vi "ExampleSubEvent.vi"(7 "error in (no error)":errorcluster, 8 "Stop Button event source":refnum<vi>, 10 "Button Array event source":refnum<vi>[](array[refnum])) -> (0 "error out":errorcluster)   [LabVIEW 2020]
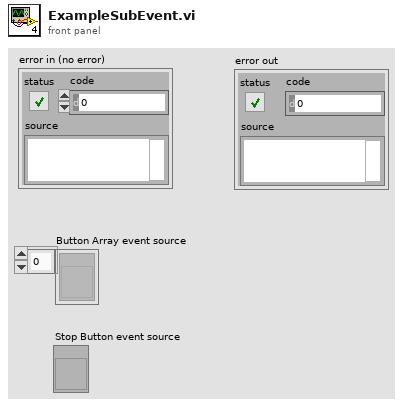
[diagram p1: front panel]
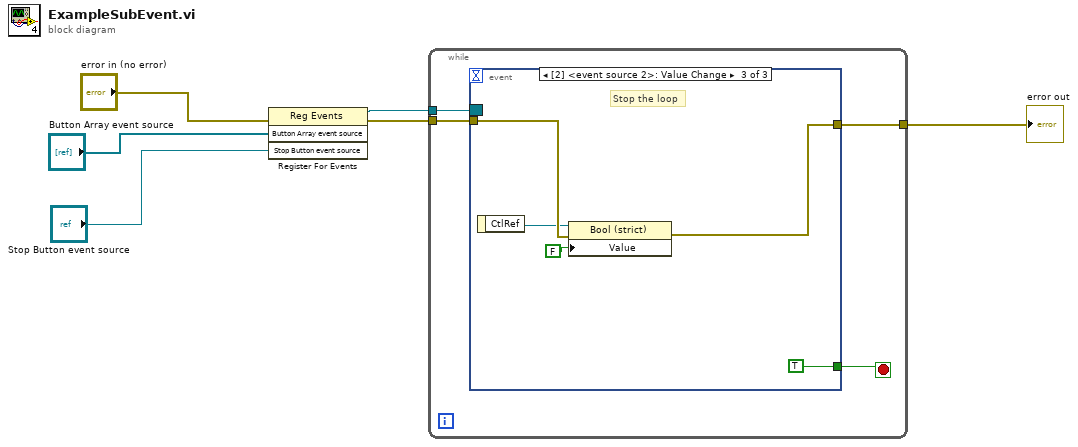
[diagram p0: block diagram]
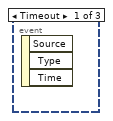
[diagram p2: hidden frame]
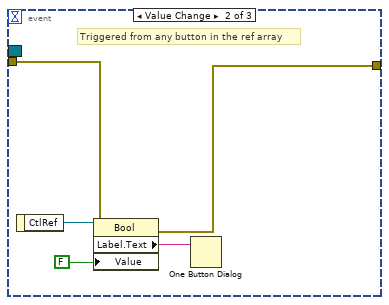
[diagram p3: hidden frame]
diagram:
  n1 = register-events(error in="error in (no error)", "Button Array event source", "Stop Button event source") -> (reference out=w6:refnum<event-registration>, error out=w5:errorcluster)  [unwired: 1 in]
  n2 = while {
    tunnel: w6 -> [w10]
    tunnel: w5 -> [w9]
    tunnel: [w8] -> w4
    stop <- w7 stop-if-true
    n3 = event shown="[2] <event source 2>: Value Change" {
      selector: w10 -> [_ _ _]
      dyn-events: _ -> [_ _ _]
      timeout: _ -> [_ _ _]
      tunnel: w9 -> [_ w12 w20]
      tunnel: [_ w11 w18] -> w8
      tunnel: [_ _ TRUE] -> w7
      event Timeout {
        n4 = event-data() -> ()  [unwired: 1 in, 3 out]
      }
      event Value Change {
        # "Triggered from any button in the ref array"
        n5 = event-data() -> ("CtlRef"=w15:refnum<vi>)  [unwired: 1 in]
        n6 = property class="Bool"(reference=w15, error in=w12, "Value"=FALSE) -> (error out=w11:errorcluster, "Label.Text"=w14:string)  [unwired: 1 out]
        n7 = One Button Dialog(message=w14) -> ()  [unwired: 1 in, 1 out]
      }
      event Value Change {
        # "Stop the loop"
        n8 = event-data() -> ("CtlRef"=w19:refnum<vi>)  [unwired: 1 in]
        n9 = property class="Bool (strict)"(reference=w19, error in=w20, "Value"=FALSE) -> (error out=w18:errorcluster)  [unwired: 1 out]
      }
    }
  }
  "error out" <- w4
